vi "setParameters.vi"(10 "Parameters":T1, 11 "ClearAberrationCommand in":refnum<class "ClearAberrationCommand.lvclass">) -> (3 "ClearAberrationCommand out":refnum<class "ClearAberrationCommand.lvclass">)   [LabVIEW 2016, in "ClearAberrationCommand.lvclass"]
uses:
  ClearAberrationCommand.lvclass
  DataTypes/Topics/CommandClearAberration.ctl
  DataTypes/Topics/Parts/CommandId.ctl
  ClearAberrationCommand.lvclass/ClearAberrationCommand.ctl
  DataTypes/Topics/M1M3SupportTopics.lvlib
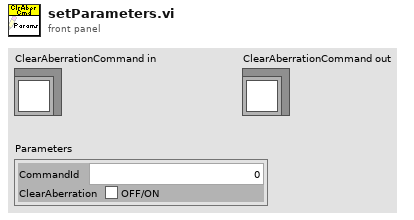
[diagram p1: front panel]
types:
  T1 = typedef "M1M3SupportTopics.lvlib/CommandClearAberration.ctl" = cluster{"CommandId":T2, "ClearAberration":bool}
  T2 = typedef "M1M3SupportTopics.lvlib/CommandId.ctl" = i32
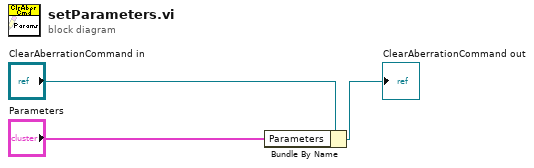
[diagram p0: block diagram]
diagram:
  n1 = Bundle By Name(cluster="ClearAberrationCommand in", "Parameters"="Parameters") -> (→"ClearAberrationCommand out":refnum<class "ClearAberrationCommand.lvclass">)
